vi "Get Instrument Type ID.vi"(8 "error in":errorcluster, 11 "session factory in":refnum<class "Session Factory.lvclass">) -> (0 "error out":errorcluster, 2 "instrument type id":string, 3 "session factory out":refnum<class "Session Factory.lvclass">)   [LabVIEW 2020, in "MeasurementLink niDMM.lvlib" / "Session Factory.lvclass"]
uses:
  Session Factory.lvclass
  Session Factory.lvclass/Session Factory.ctl
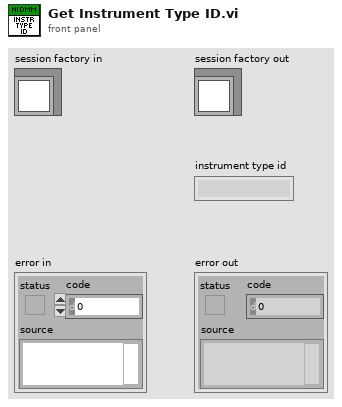
[diagram p1: front panel]
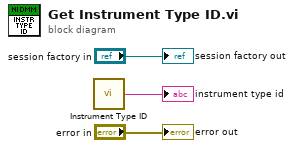
[diagram p0: block diagram]
diagram:
  n1 = call "Instrument Type ID.vi"() -> ("instrument type id"=→"instrument type id":string)  [unwired: 5 in]
  "error out" <- "error in"
  "session factory out" <- "session factory in"
